vi "UpdateRegisterFile.vi"(8 "error in (no error)":errorcluster, 9 "eI2Cflags":T1 caption="I2C Flags" items=["None"=0, "START"=2, "REPEATED START"=3, "STOP"=4, "START AND STOP"=6], 10 "Buffer":u8[](array[numeric]), 11 "I2COUSBSim in":refnum<class "I2COUSBSim.lvclass">) -> (0 "error out":errorcluster, 3 "I2COUSBSim out":refnum<class "I2COUSBSim.lvclass">)   [LabVIEW 2020, in "I2COUSB.lvlib" / "I2COUSBSim.lvclass"]
uses:
  I2COUSBSim.lvclass
  II2COUSB/II2COUSB/I2CFlags.ctl
  I2COUSBSim.lvclass/I2COUSBSim.ctl
  II2COUSB/II2COUSB/II2COUSB.lvclass
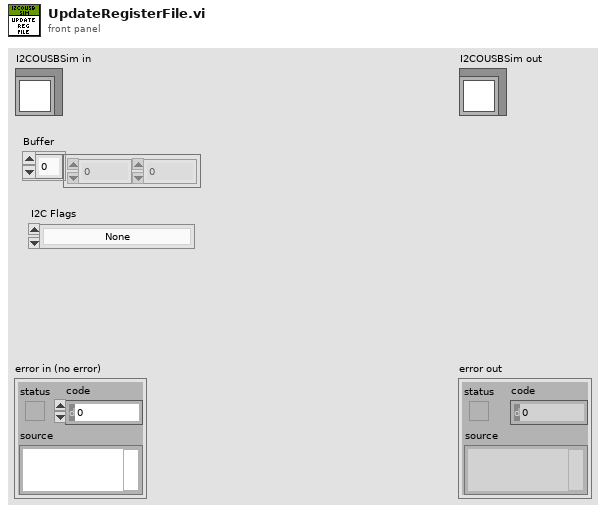
[diagram p1: front panel]
types:
  T1 = typedef "II2COUSB.lvlib/II2COUSB.lvclass/I2CFlags.ctl" = u8
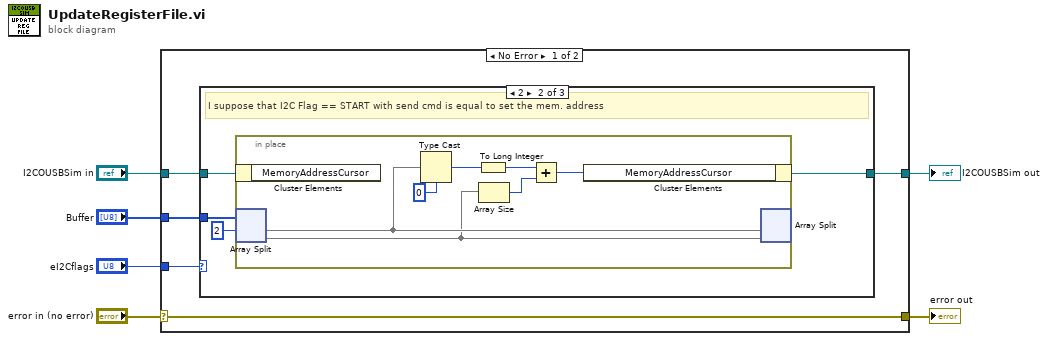
[diagram p0: block diagram]
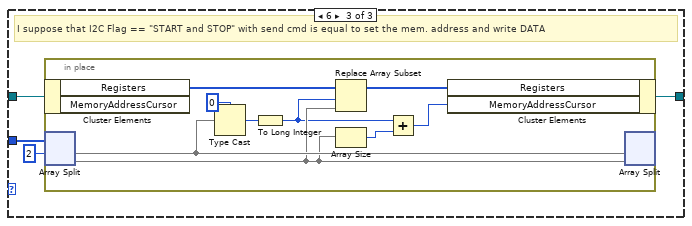
[diagram p3: hidden frame]
diagram:
  n1 = case shown="No Error" "error in (no error)" {
    selector: "error in (no error)" -> [w11 w38]
    tunnel: [w11 w38] -> w5
    tunnel: [w7 w37] -> w3
    tunnel: "I2COUSBSim in" -> [w8 w37]
    tunnel: "eI2Cflags" -> [w10 _]
    tunnel: "Buffer" -> [w9 _]
    frame No Error {
      n2 = case shown="2" w10 {
        tunnel: w9 -> [_ w15 w26]
        tunnel: w8 -> [w12 w16 w27]
        tunnel: [w12 w13 w24] -> w7
        frame Default {
          # "I suppose that others I2C Flag settings are not used wiith send cmd. So i nothing to do"
        }
        frame 2 {
          # "I suppose that I2C Flag == START with send cmd is equal to set the mem. address"
          n3 = in-place {
            n4 = in-place-cluster #1(w16) -> ()  [unwired: 1 out]
            n5 = in-place-split #2(w15, 2) -> (w21:u8[], w20:u8[])
            n6 = Type Cast(type=u16 0, x=w21) -> (*(type *) &x=w22:u16)
            n7 = To Long Integer(number=w22) -> (32bit integer=w19:i32)
            n8 = Array Size(array=w20) -> (size(s)=w18:i32)
            n9 = Add(x=w19, y=w18) -> (x+y=w17:i32)
            n10 = in-place-cluster #1("MemoryAddressCursor"=w17) -> (w13:refnum<class "I2COUSBSim.lvclass">)
            n11 = in-place-split #2(w21, w20) -> ()  [unwired: 2 out]
          }
        }
        frame 6 {
          # "I suppose that I2C Flag == \"START and STOP\" with send cmd is equal to set the mem. address and write DATA"
          n12 = in-place {
            n13 = in-place-cluster #3(w27) -> ("Registers"=w36:u8[])  [unwired: 1 out]
            n14 = in-place-split #4(w26, 2) -> (w32:u8[], w31:u8[])
            n15 = Type Cast(type=u16 0, x=w32) -> (*(type *) &x=w33:u16)
            n16 = To Long Integer(number=w33) -> (32bit integer=w30:i32)
            n17 = Replace Array Subset(array=w36, new element=w31, index=w30) -> (w35:u8[])
            n18 = Array Size(array=w31) -> (size(s)=w29:i32)
            n19 = Add(x=w30, y=w29) -> (x+y=w28:i32)
            n20 = in-place-cluster #3("Registers"=w35, "MemoryAddressCursor"=w28) -> (w24:refnum<class "I2COUSBSim.lvclass">)
            n21 = in-place-split #4(w32, w31) -> ()  [unwired: 2 out]
          }
        }
      }
    }
    frame Error {
    }
  }
  "error out" <- w5
  "I2COUSBSim out" <- w3
